vi "FlatToRichnidevice_grpc_EnumerateDevicesRequest.vi"(5 "OutputClusterType":T1, 11 "InputCluster":T2) -> (3 "OutputCluster":T1)   [LabVIEW 2021, in "NI DAQmx_server.lvlib"]
uses:
  nidevice_grpc_EnumerateDevicesRequest_Flat.ctl
  nidevice_grpc_EnumerateDevicesRequest.ctl
  NI DAQmx_server.lvlib
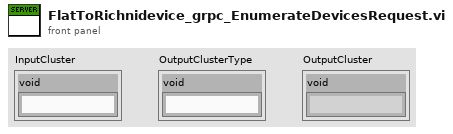
[diagram p1: front panel]
types:
  T1 = typedef "NI DAQmx_server.lvlib/nidevice_grpc_EnumerateDevicesRequest.ctl" = cluster{"void":string}
  T2 = typedef "NI DAQmx_server.lvlib/nidevice_grpc_EnumerateDevicesRequest_Flat.ctl" = cluster{"void":string}
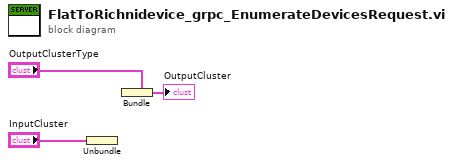
[diagram p0: block diagram]
diagram:
  n1 = Unbundle "Unbundle"("InputCluster") -> ()  [unwired: 1 out]
  n2 = Bundle "Bundle"(cluster="OutputClusterType") -> (→"OutputCluster":T1)  [unwired: 1 in]
